vi "FILE_DIALOG 2016.vi"(0 "flow_slope_IN":dbl=51.35 format="%.2f", 1 "pressure_slope_IN":dbl=23.33 format="%.2f", 2 "DHT_Pressure_In":dbl=1.5 format="%.2f", 4 "string_pot_slope_IN":dbl=1.5 format="%.2f", 5 "Descriptions":string[](array[string]), 6 "DHT_Pressure_In Offset":dbl=1.5 format="%.2f", 7 "error in (no error)":errorcluster, 8 "start path":path=path "D:/Cascade/Data/Output Files", 9 "Sensor Cluster":T1, 11 "Aux1_In":dbl=1.5 format="%.2f", 14 "Array in":refnum<k24>[](array[refnum]), 17 "Aux2_In":dbl=1.5 format="%.2f", 19 "Aux3_In":dbl=1.5 format="%.2f") -> (12 "Output path":path, 13 "Sensor Cluster 2":T1, 15 "exists":bool, 16 "Array out":refnum<k24>[](array[refnum]), 20 "flow_slope_OUT":dbl=51.35 format="%.2f", 21 "pressure_slope_OUT":dbl=732.5347533511234 format="%.2f", 23 "Record Output Slopes to  Record File":path, 24 "string_pot_slope_OUT":dbl=1.5 format="%.2f", 25 "Record Output Slopes for slopes.csv File":path, 27 "error out":errorcluster)   [LabVIEW 2016]
uses:
  C:/Program Files/National Instruments/LabVIEW 2016/vi.lib/ULx/ULx_LV.dll
  Program Files/National Instruments/LabVIEW 2016/vi.lib/ULx/ULx_LV.dll
  controls/MCC DAQ Readings.ctl
  <userlib>/_OpenG.lib/file/file.llb/Strip Path - Traditional__ogtk.vi
  <userlib>/_OpenG.lib/file/file.llb/Build Path - Traditional__ogtk.vi
  <userlib>/_OpenG.lib/file/file.llb/File Exists - Scalar__ogtk.vi
panel:
  out "Loop Counter":i32
  out "cal_completed":bool
  out "new_or _prev_file_selected":bool
  in  "calibrate_KPRO":bool
  in  "previous_file":bool
  in  "new_file":bool
  in  "OK Button":bool
  # "For a new file, open the  directory with the new profile ID name and click 'Current Folder' to use that folder.  For a previous file, click on the ProfileID_KPROCumulative.csv file"
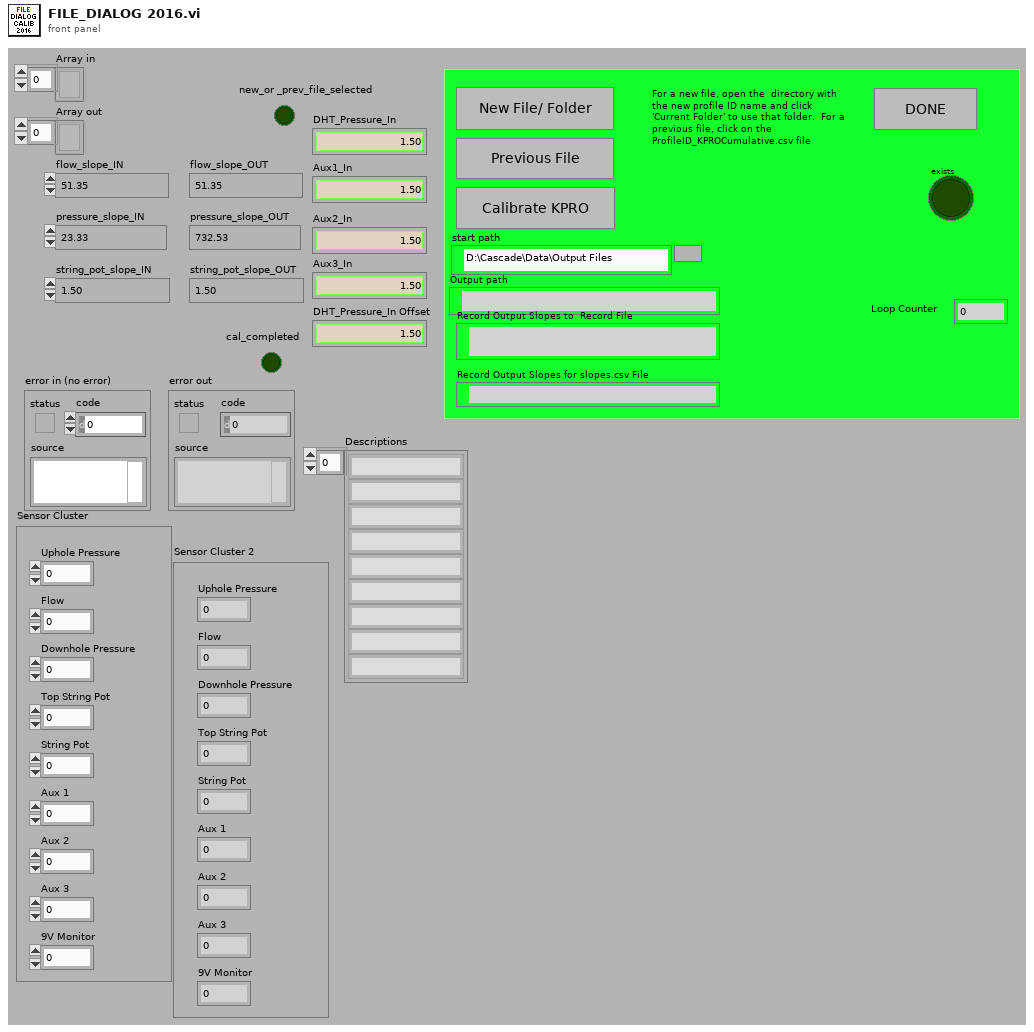
[diagram p1: front panel]
types:
  T1 = typedef "MCC DAQ Readings.ctl" = cluster{"Uphole Pressure":dbl, "Flow":dbl, "Downhole Pressure":dbl, "Top String Pot":dbl, "String Pot":dbl, "Aux 1":dbl, "Aux 2":dbl, "Aux 3":dbl, "9V Monitor":dbl}
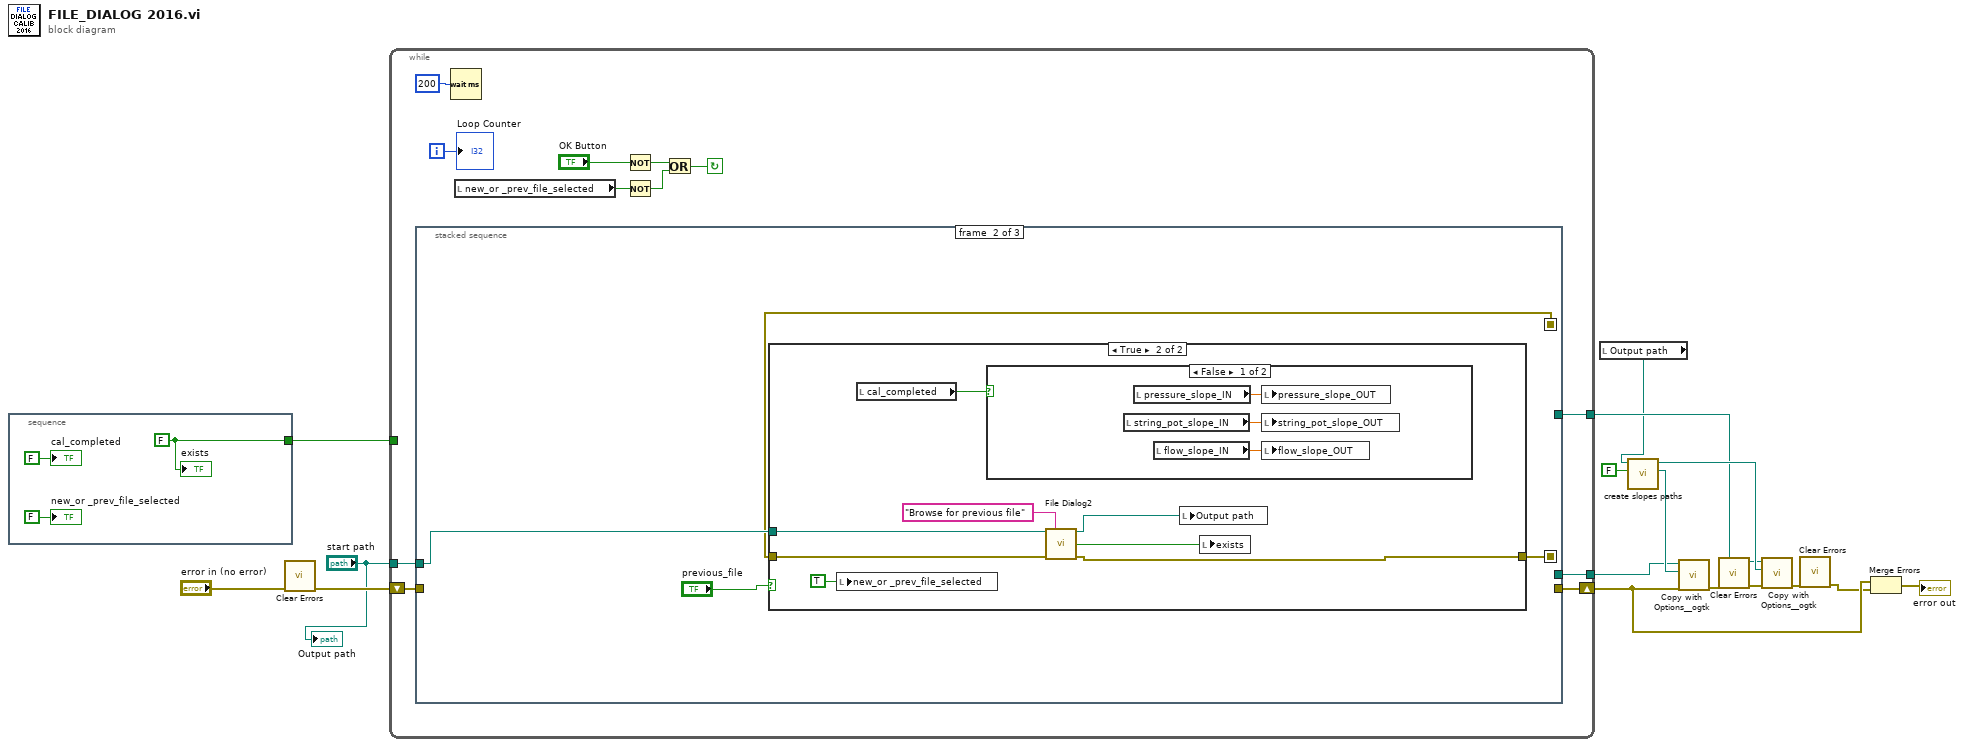
[diagram p0: block diagram]
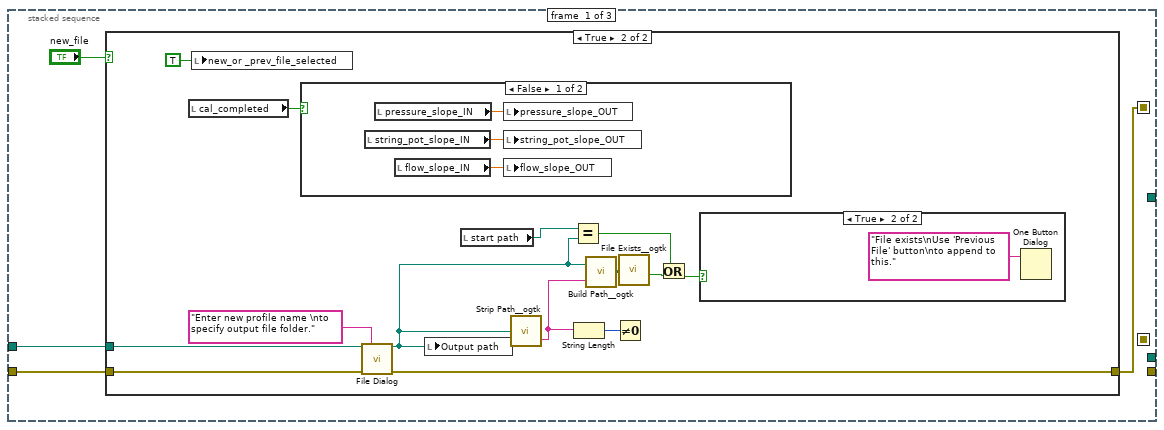
[diagram p2: hidden frame]
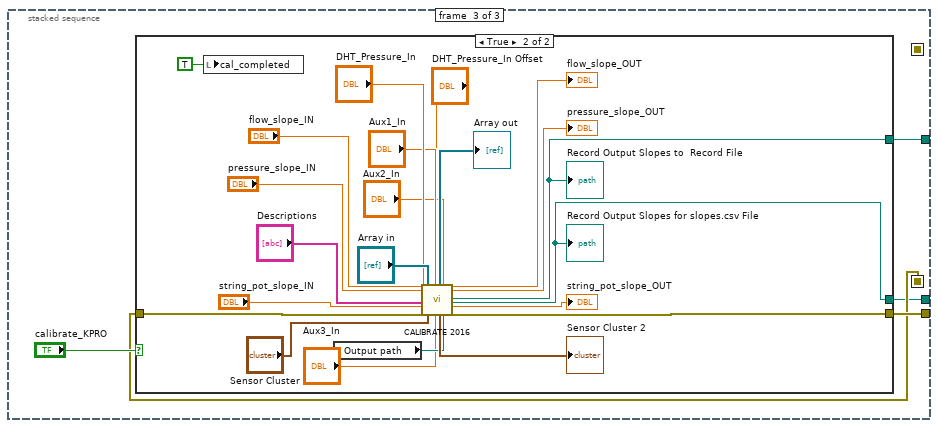
[diagram p8: hidden frame]
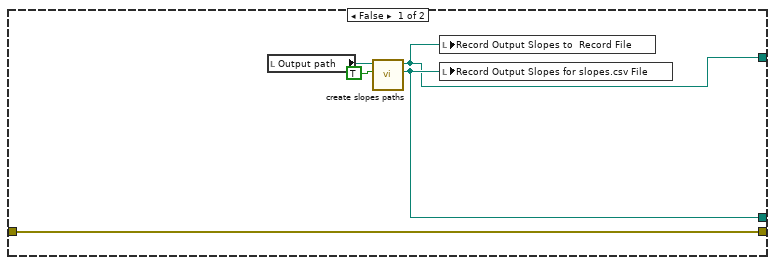
[diagram p9: hidden frame]
diagram:
  n1 = stacked-sequence {
    tunnel: [w19] -> w16
    frame #0 {
      w19 = FALSE ("exists")
      "exists" <- w19
      "new_or _prev_file_selected" <- FALSE ("new_or _prev_file_selected")
      "cal_completed" <- FALSE ("cal_completed")
    }
  }
  n2 = call <vilib>:"Clear Errors.vi"("error in (no error)"="error in (no error)") -> ("error out"=w14:errorcluster)  [unwired: 5 in, 1 out]
  n3 = while {
    shift-left: w14 -> [w28]
    shift-right: [w27] -> w4
    tunnel: "start path" -> [w29]
    tunnel: w16 -> [_]
    tunnel: [w21] -> w8
    tunnel: [w20] -> w7
    i -> [w22]
    stop <- w26 continue-if-true
    n4 = stacked-sequence {
      seq-local: [w32 _ _] -> [_ w56 _]
      seq-local: [_ w55 _] -> [_ _ w73]
      tunnel: w29 -> [w34 w57 _]
      tunnel: w28 -> [w33 _ _]
      tunnel: [_ _ w74] -> w27
      tunnel: [_ _ w72] -> w21
      tunnel: [_ _ w71] -> w20
      frame #0 {
        n5 = case shown="True" "new_file" {
          tunnel: w34 -> [_ w47]
          tunnel: w33 -> [w36 w46]
          tunnel: [w36 w45] -> w32
          frame False {
          }
          frame True {
            n6 = local read "cal_completed"() -> (w49:bool)
            n7 = local write "new_or _prev_file_selected"(TRUE ("new_or _prev_file_selected")) -> ()
            n8 = case shown="False" w49 {
              frame False {
                n9 = local read "string_pot_slope_IN"() -> (w51:dbl)
                n10 = local read "pressure_slope_IN"() -> (w52:dbl)
                n11 = local read "flow_slope_IN"() -> (w53:dbl)
                n12 = local write "pressure_slope_OUT"(w52) -> ()
                n13 = local write "string_pot_slope_OUT"(w51) -> ()
                n14 = local write "flow_slope_OUT"(w53) -> ()
              }
              frame True {
              }
            }
            n15 = call "File Dialog"("start path"=w47, "prompt"="Enter new profile name \nto specify output file folder.", "error in"=w46) -> ("selected path"=w38:path, "error out"=w45:errorcluster)  [unwired: 9 in, 2 out]
            n16 = local write "Output path"(w38) -> ()
            n17 = local read "start path"() -> (w39:path)
            n18 = call-poly <userlib>:"Strip Path__ogtk.vi"("path"=w38) -> ("name"=w42:string)  [unwired: 1 out]
            n19 = Equal?(x=w39, y=w38) -> (x = y?=w37:bool)
            n20 = String Length(string=w42) -> (length=w40:i32)
            n21 = call-poly <userlib>:"Build Path__ogtk.vi"("name or relative path"=w42, "base path"=w38) -> ("appended path"=w43:path)
            n22 = Not Equal To 0?(x=w40) -> ()  [unwired: 1 out]
            n23 = call-poly <userlib>:"File Exists__ogtk.vi"("file path"=w43) -> ("exists"=w44:bool)  [unwired: 6 in, 1 out]
            n24 = Or(x=w37, y=w44) -> (x .or. y?=w41:bool)
            n25 = case shown="True" w41 {
              frame False {
              }
              frame True {
                n26 = One Button Dialog(message="File exists\nUse 'Previous File' button\nto append to this.") -> ()  [unwired: 1 in, 1 out]
              }
            }
          }
        }
      }
      frame #1 {
        n27 = case shown="True" "previous_file" {
          tunnel: w57 -> [_ w64]
          tunnel: w56 -> [w59 w61]
          tunnel: [w59 w60] -> w55
          frame False {
          }
          frame True {
            n28 = local write "new_or _prev_file_selected"(TRUE ("new_or _prev_file_selected")) -> ()
            n29 = local read "cal_completed"() -> (w66:bool)
            n30 = case shown="False" w66 {
              frame False {
                n31 = local read "string_pot_slope_IN"() -> (w68:dbl)
                n32 = local read "pressure_slope_IN"() -> (w69:dbl)
                n33 = local read "flow_slope_IN"() -> (w70:dbl)
                n34 = local write "pressure_slope_OUT"(w69) -> ()
                n35 = local write "string_pot_slope_OUT"(w68) -> ()
                n36 = local write "flow_slope_OUT"(w70) -> ()
              }
              frame True {
              }
            }
            n37 = call "File Dialog2"("start path"=w64, "prompt"="Browse for previous file", "error in"=w61) -> ("selected path"=w63:path, "exists"=w62:bool, "error out"=w60:errorcluster)  [unwired: 9 in, 1 out]
            n38 = local write "Output path"(w63) -> ()
            n39 = local write "exists"(w62) -> ()
          }
        }
      }
      frame #2 {
        n40 = case shown="True" "calibrate_KPRO" {
          tunnel: w73 -> [w80 w99]
          tunnel: [w80 w98] -> w74
          tunnel: [w77 w87] -> w72
          tunnel: [w76 w86] -> w71
          frame False {
            n41 = local read "Output path"() -> (w79:path)
            n42 = call "create slopes paths.vi"("Strip Path"=TRUE, "Path"=w79) -> ("Record Output Slopes for slopes.csv File"=w77:path, "Record Output Slopes to  Record File"=w76:path)  [unwired: 8 in]
            n43 = local write "Record Output Slopes to  Record File"(w76) -> ()
            n44 = local write "Record Output Slopes for slopes.csv File"(w77) -> ()
          }
          frame True {
            n45 = local write "cal_completed"(TRUE ("cal_completed")) -> ()
            n46 = local read "Output path"() -> (w88:path)
            n47 = call "CALIBRATE 2016.vi"("flow_slope_IN"="flow_slope_IN", "pressure_slope_IN"="pressure_slope_IN", "DHT_Pressure_In"="DHT_Pressure_In", "Descriptions"="Descriptions", "string_pot_slope_IN"="string_pot_slope_IN", "DHT_Pressure_In Offset"="DHT_Pressure_In Offset", "error in (no error)"=w99, "Array in"="Array in", "Sensor Cluster"="Sensor Cluster", "Aux1_In"="Aux1_In", "Aux3_In"="Aux3_In", "Aux2_In"="Aux2_In", "Path"=w88) -> ("Array out"=→"Array out":refnum<k24>[], "Sensor Cluster 2"=→"Sensor Cluster 2":T1, "flow_slope_OUT"=→"flow_slope_OUT":dbl, "pressure_slope_OUT"=→"pressure_slope_OUT":dbl, "Record Output Slopes to  Record File"=w86:path, "Record Output Slopes for slopes.csv File"=w87:path, "string_pot_slope_OUT"=→"string_pot_slope_OUT":dbl, "error out"=w98:errorcluster)  [unwired: 7 in]
            "Record Output Slopes to  Record File" <- w86
            "Record Output Slopes for slopes.csv File" <- w87
          }
        }
      }
    }
    n48 = Wait (ms)(milliseconds to wait=u32 200) -> ()  [unwired: 1 out]
    n49 = local read "new_or _prev_file_selected"() -> (w24:bool)
    n50 = Not(x="OK Button") -> (.not. x?=w25:bool)
    n51 = Not(x=w24) -> (.not. x?=w23:bool)
    n52 = Or(x=w25, y=w23) -> (x .or. y?=w26:bool)
    "Loop Counter" <- w22
  }
  n53 = local read "Output path"() -> (w6:path)
  n54 = call "create slopes paths.vi"("Strip Path"=FALSE, "Path"=w6) -> ("Record Output Slopes for slopes.csv File"=w11:path, "Record Output Slopes to  Record File"=w13:path)  [unwired: 8 in]
  n55 = call <userlib>:"Copy with Options__ogtk.vi"("error in (no error)"=w4, "target path"=w11, "source path"=w8) -> ("error out"=w12:errorcluster)  [unwired: 7 in, 1 out]
  n56 = call <vilib>:"Clear Errors.vi"("error in (no error)"=w12) -> ("error out"=w2:errorcluster)  [unwired: 5 in, 1 out]
  n57 = call <userlib>:"Copy with Options__ogtk.vi"("error in (no error)"=w2, "target path"=w13, "source path"=w7) -> ("error out"=w9:errorcluster)  [unwired: 7 in, 1 out]
  n58 = call <vilib>:"Clear Errors.vi"("error in (no error)"=w9) -> ("error out"=w3:errorcluster)  [unwired: 5 in, 1 out]
  n59 = Merge Errors(w4, w3) -> (→"error out":errorcluster)
  "Output path" <- "start path"
